vi "RealSense_HelloWorld_On-Chip-Calibration4.vi"() -> ()   [LabVIEW 2017]
doc: "Simple Demo showing how to connect a RealSense Camera to stream COLOR and DEPTH from the stereo camera of a D4xx series camera."
uses:
  healthCheck2.ctl
  libRealSense3.lvlib
panel:
  out "frame time, ms":i64=25
  in  "stop":bool=TRUE
  in  "Use 256x144 for On-Chip Calibration!":u16(ring) items=["256 x 144 @90fps", "424 x 240 @6fps", "424 x 240 @15fps", "424 x 240 @30fps", "424 x 240 @60fps", "424 x 240 @90fps", "480 x 270 @6fps", "480 x 270 @15fps", "480 x 270 @30fps", "480 x 270 @60fps", "480 x 270 @90fps", "640 x 360 @6fps", "640 x 360 @15fps", "640 x 360 @30fps", "640 x 360 @60fps", "640 x 360 @90fps", "640 x 480 @6fps", "640 x 480 @15fps", "640 x 480 @30fps", "640 x 480 @60fps", "640 x 480 @90fps", "848 x 100 @100fps", "848 x 480 @6fps", "848 x 480 @15fps", "848 x 480 @30fps", "848 x 480 @60fps", "848 x 480 @90fps", "1280 x 720 @6fps", "1280 x 720 @15fps", "1280 x 720 @30fps", "1920 x 1080 @15fps", "1920 x 1080 @25fps"]
  in  "Tab Control":T1(tab)
  in  "Depth Presets":T2(ring)=enum."High Accuracy"
  out "Error":bool
  out "Error":bool
  out "AngleX, deg":dbl=-6.76056287473476 format="%.2f"
  out "AngleY, deg":dbl=0.9024890486254136 format="%.2f"
  out "Subpixel, pix":dbl=0.13037986141603491 format="%_3g"
  out "rms error, mm":dbl=1.176758916205707 format="%_3g"
  out "Fill factor (%)":dbl=67.74631076388889 format="%_4g"
  in  "Old / New":bool=TRUE
  in  "SelfCal":bool
  in  "Burn":bool
  out "Healthcheck":T3=0.01235621701925993 scale=0.0..1.8
  in  "laser on/off":bool
  in  "Laser Power,\n mW":sgl=150.0 min=0 max=360
  in  "Gain":sgl=16.0 min=16 max=248
  out "RGB image":picture
  in  "autoexposure":bool
  in  "Exposure,us":sgl=13000.0 min=20 max=1660000
  in  "Tare":bool
  out "Cal Error":string
  in  "Ground Truth, mm":dbl=544.0 format="%.1f"
  out "Measured Z, mm":dbl=543.8435973412348 format="%.1f"
  out "accuracy, %":dbl=-0.02875048874359553 format="%.2f"
  out "Depth map":dbl[][](graph)
  out "OldCalibrationTable":u64=1750951606032
  out "NewCalibrationTable":u64=1750951606320
  in  "Recover Factory Cal.\n(Will stop program)":bool
  in  "Auto Depth Preset\n(5 sec slower)":bool
  in  "A-factor":dbl=0.2
  in  "Calibration Mode":u16(ring) items=["Intrinsic", "Extrinsic"]
  in  "Linux/Windows":u16(ring) items=["Linux+Windows", "Windows Faster"]
  in  "averaging(<30)":u16=10
  in  "Maxstep(5-30)":u16=20
  in  "Accuracy target":u8(ring) items=["Very High (0.025%)", "High (0.05%)", "Medium  (0.1%)", "Low (0.2%)"]
  in  "Self-Calibration Speed":T4(ring)=enum."Fast (Default)"
  out "Camera initialization results":T5={"camera name"="Intel RealSense D435I", "camera S/N"="834412070342", "F/W"="05.12.01.00", "Sensor name"="Stereo Module", "api_version"=23201, "rscontext"=1750951079632, "device_list"=1750948995696, "device count"=1, "Dev out"=1751051540560, "sensor_list"=1750951514688, "sensor count"=3, "Sensor out"=1750945215376}
  out "init error":string="\rNo Error\rNo Error\rNo Error\rNo Error\rNo Error\rNo Error\rNo Error\r\rNo Error\rNo Error"
  out "Config error":string="No Error\rNo Error"
  out "Start Error":string="No Error\rNo Error\rNo Error"
  out "Capture1 Error":string="No Error"
  out "Capture2 error":string="No Error"
  out "Close Error":string="No Error\rNo Error\rNo Error\rNo Error"
  out "release frame error":string="No Error"
  out "Stereo baseline, mm":dbl=49.90683364868164
  out "Intrinsics":T6={"width"=256, "height"=144, "fps"=90, "Profile"=1750952767112, "ppx"=126.45603, "ppy"=71.40294, "fx"=131.32307, "fy"=131.32307, "model"=4}
  # "RealSense Hello World: On-Chip Calibration & Tare"
  # "This demo shows how to connect a RealSense D4xx Stereo Depth Camera, and stream the Monochrome (left) and a DEPTH MAP, and then run on-chip 1. self-calibration to improve depth noise, and 2. Tare to improve accuracy."
  # "MONOCHROME"
  # "ZOOMED (20%) DEPTH MAP"
  # "20-1660000"
  # "Fail-Safe"
  # "16-248"
  # "Point to Flat Wall. Enter the Ground Truth value, and then press Tare. Select \"high accuracy\" Depth Preset before running)"
  # "SELF-CAL \n(DEPTH RMS NOISE)"
  # "Toggle\nCalib."
  # "BURN\n(to ASIC)"
  # "TARE\n(SCALE)"
  # "Point to scene with more than 50% valid depth. Press Self-Cal."
  # "0-360"
  # "Burn after each Tare or Self-Cal."
  # "Common Calibration Settings"
  # "Camera Settings"
  # "For Tare when using \"high accuracy\" depth preset, we recommend using A-factor = 0.2\nFor \"high density\" we recommend A=0.1"
  # "Tare Settings"
  # "Self-Calibration Settings"
  # "The \"speed\" defines the search range. Use \"Fast\" by default, and if you get \"out of range\" error, then try \"slow\""
  # "Use averaging=10, and MaxSteps=20, and Accuracy=Very High for best results. Be sure to use High Accuracy Depth preset or Auto Preset (which will be ~5 seconds slower)"
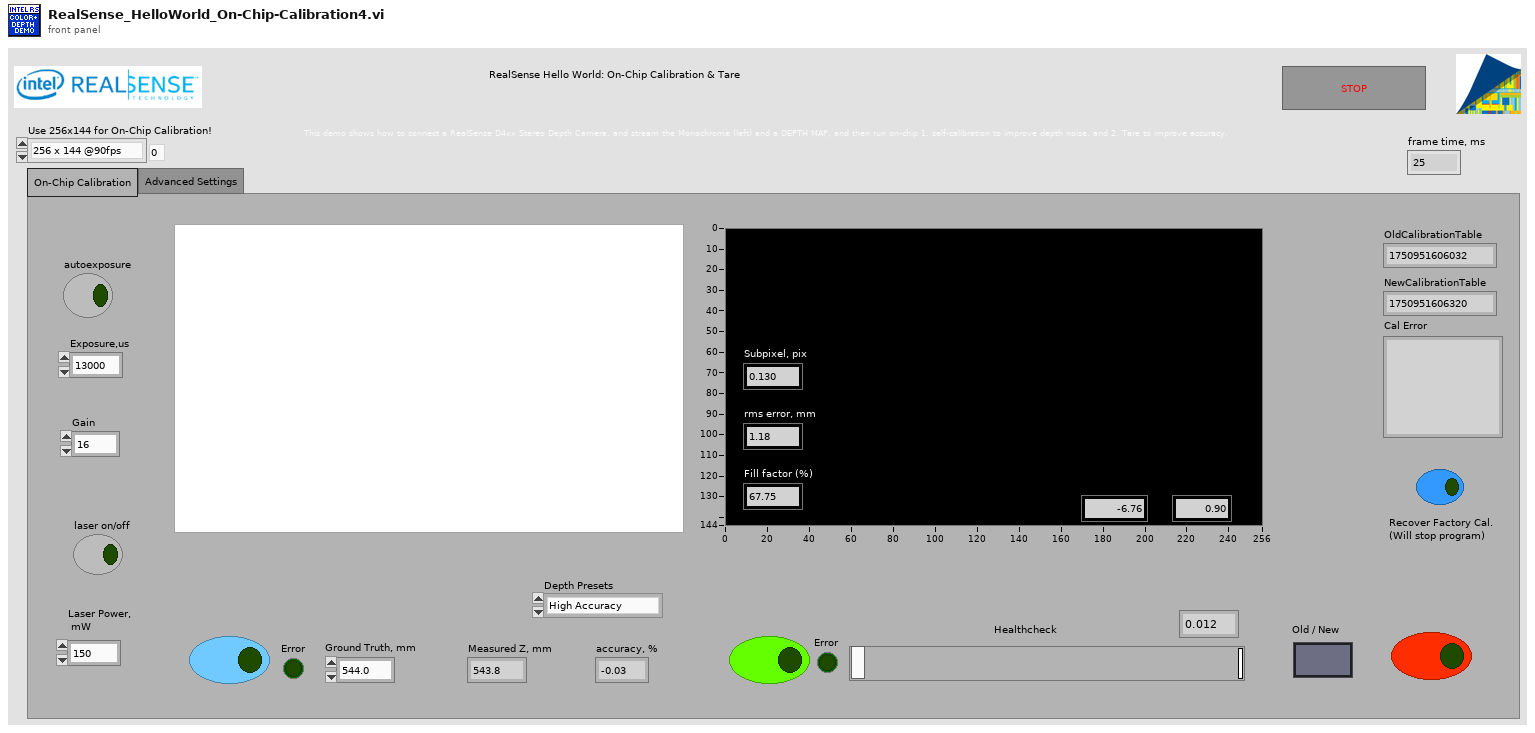
[diagram p1: front panel]
types:
  T1 = enum32{"On-Chip Calibration", "Advanced Settings"}
  T2 = enum16{"Original", "High Density", "Medium Density", "High Accuracy", "Hand", "Short Range", "Flat wall"}
  T3 = typedef "libRealSense3.lvlib/healthCheck2.ctl" = dbl
  T4 = enum16{"Very Fast", "Fast (Default)", "Medium", "Slow", "White Wall"}
  T5 = cluster{"camera name":string, "camera S/N":string, "F/W":string, "Sensor name":string, "api_version":i32, "rscontext":u64, "device_list":u64, "device count":i32, "Dev out":u64, "sensor_list":u64, "sensor count":i32, "Sensor out":u64}
  T6 = cluster{"width":i32, "height":i32, "fps":i32, "Profile":u64, "ppx":sgl, "ppy":sgl, "fx":sgl, "fy":sgl, "model":u32}
  T7 = cluster{"depthUnits":u32, "depthClampMin":u32, "depthClampMax":u32, "disparityMultiplier":u32, "disparityShift":u32}
  T8 = enum16{"Depth", "Color (ext.)", "Color (left) ", "IR Left", "IR Right", "IR Left (Y16)", "IR Right (Y16)"}
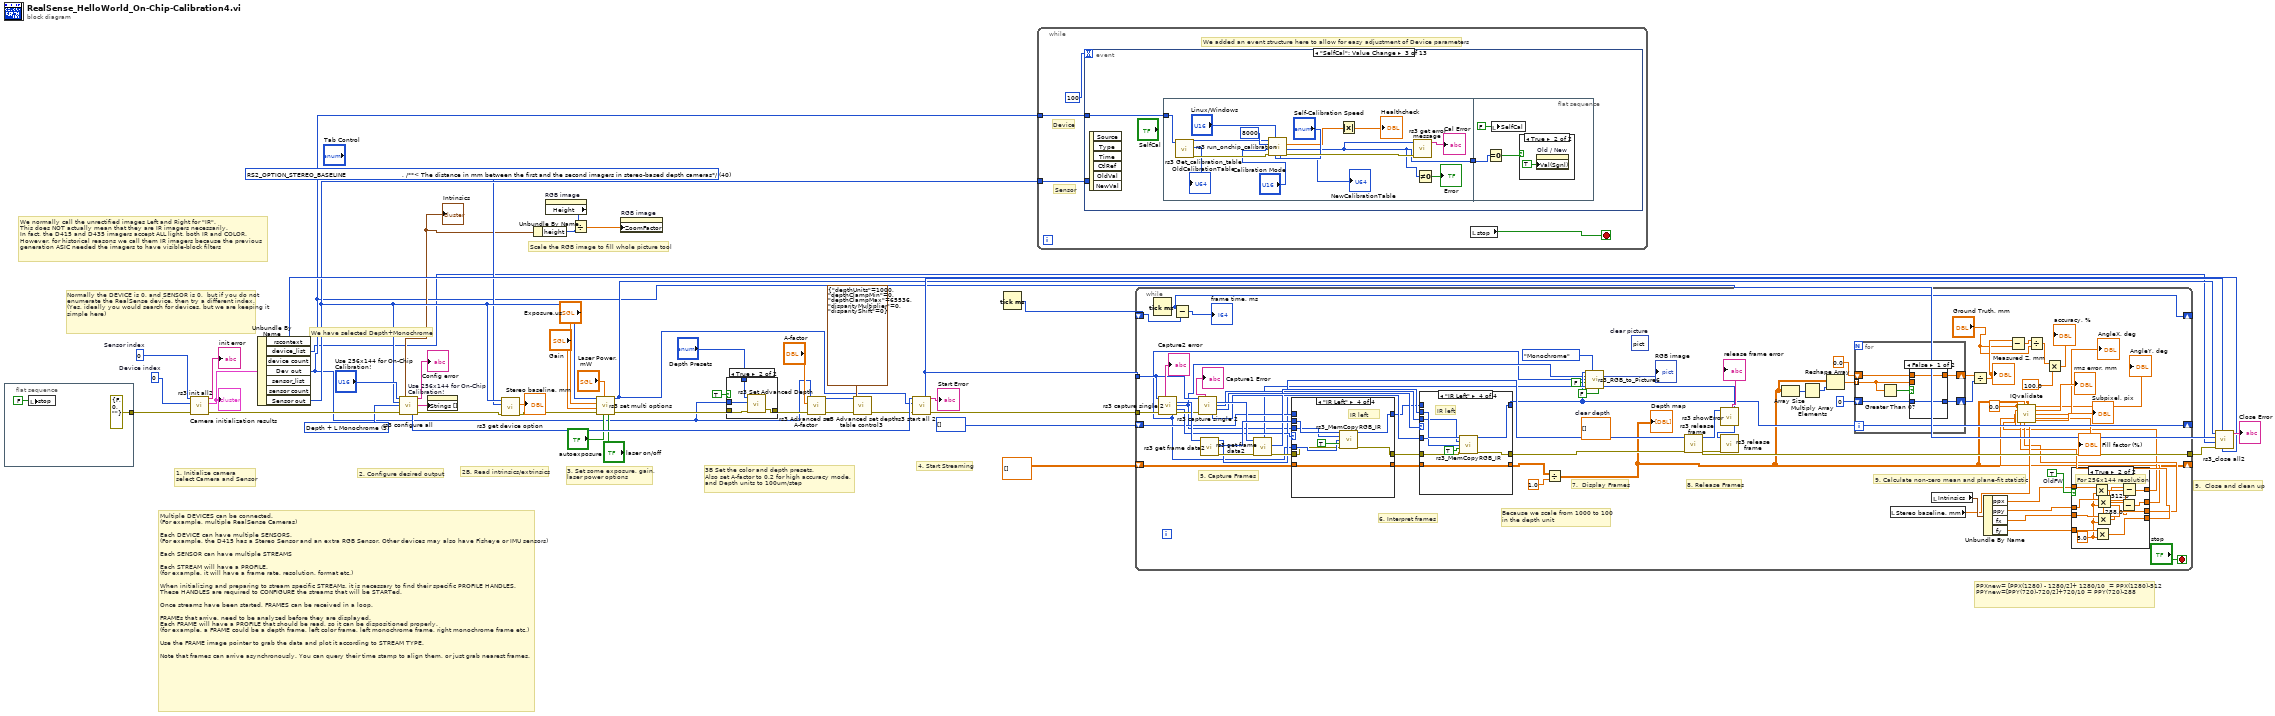
[diagram p0: block diagram]
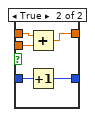
[diagram p4: hidden frame]
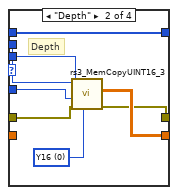
[diagram p6: hidden frame]
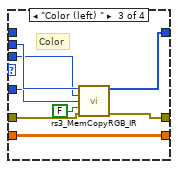
[diagram p7: hidden frame]
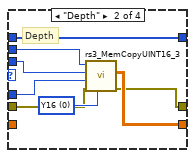
[diagram p9: hidden frame]
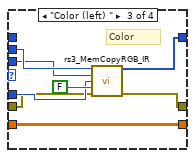
[diagram p10: hidden frame]
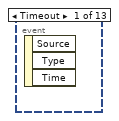
[diagram p11: hidden frame]
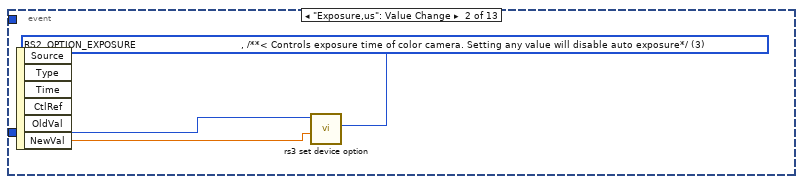
[diagram p12: hidden frame]
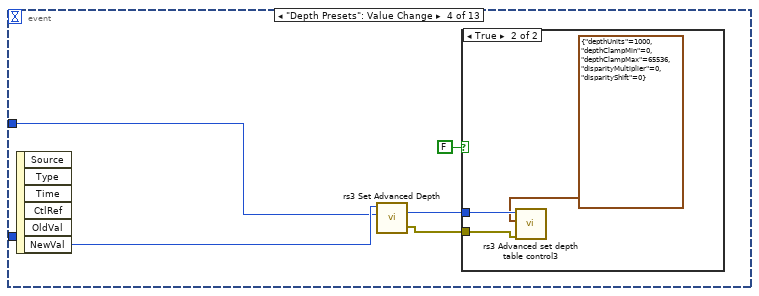
[diagram p14: hidden frame]
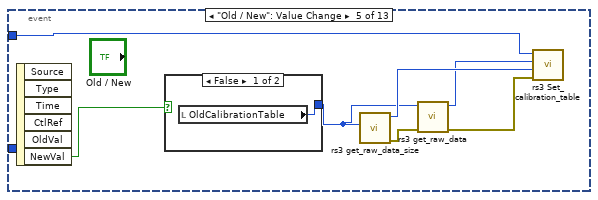
[diagram p16: hidden frame]
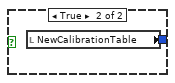
[diagram p17: hidden frame]
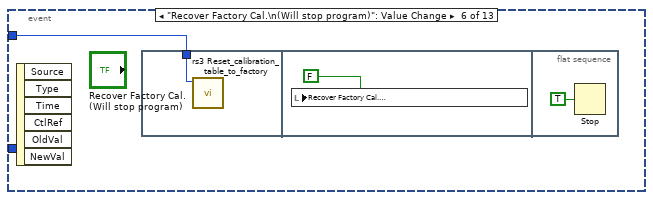
[diagram p18: hidden frame]
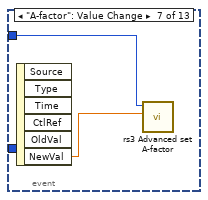
[diagram p19: hidden frame]
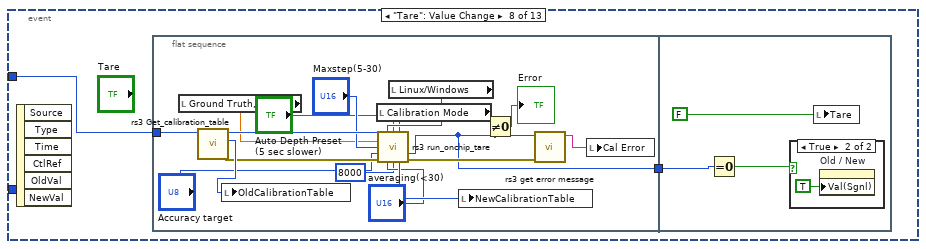
[diagram p20: hidden frame]
diagram:
  w14 = u16 40 items=["    RS2_OPTION_BACKLIGHT_COMPENSATION                     , /**< Enable / disable color backlight compensation*/", "    RS2_OPTION_BRIGHTNESS                                 , /**< Color image brightness*/", "    RS2_OPTION_CONTRAST                                   , /**< Color image contrast*/", "    RS2_OPTION_EXPOSURE                                   , /**< Controls exposure time of color camera. Setting any value will disable auto exposure*/", "    RS2_OPTION_GAIN                                       , /**< Color image gain*/", "    RS2_OPTION_GAMMA                                      , /**< Color image gamma setting*/", "    RS2_OPTION_HUE                                        , /**< Color image hue*/", "    RS2_OPTION_SATURATION                                 , /**< Color image saturation setting*/", "    RS2_OPTION_SHARPNESS                                  , /**< Color image sharpness setting*/", "    RS2_OPTION_WHITE_BALANCE                              , /**< Controls white balance of color image. Setting any value will disable auto white balance*/", "    RS2_OPTION_ENABLE_AUTO_EXPOSURE                       , /**< Enable / disable color image auto-exposure*/", "    RS2_OPTION_ENABLE_AUTO_WHITE_BALANCE                  , /**< Enable / disable color image auto-white-balance*/", "    RS2_OPTION_VISUAL_PRESET                              , /**< Provide access to several recommend sets of option presets for the depth camera */", "    RS2_OPTION_LASER_POWER                                , /**< Power of the F200 / SR300 projector, with 0 meaning projector off*/", "    RS2_OPTION_ACCURACY                                   , /**< Set the number of patterns projected per frame. The higher the accuracy value the more patterns projected. Increasing the number of patterns help to achieve better accuracy. Note that this c", "    RS2_OPTION_MOTION_RANGE                               , /**< Motion vs. Range trade-off, with lower values allowing for better motion sensitivity and higher values allowing for better depth range*/", "    RS2_OPTION_FILTER_OPTION                              , /**< Set the filter to apply to each depth frame. Each one of the filter is optimized per the application requirements*/", "    RS2_OPTION_CONFIDENCE_THRESHOLD                       , /**< The confidence level threshold used by the Depth algorithm pipe to set whether a pixel will get a valid range or will be marked with invalid range*/", "    RS2_OPTION_EMITTER_ENABLED                            , /**< Laser Emitter enabled */", "    RS2_OPTION_FRAMES_QUEUE_SIZE                          , /**< Number of frames the user is allowed to keep per stream. Trying to hold-on to more frames will cause frame-drops.*/", "    RS2_OPTION_TOTAL_FRAME_DROPS                          , /**< Total number of detected frame drops from all streams */", "    RS2_OPTION_AUTO_EXPOSURE_MODE                         , /**< Auto-Exposure modes: Static, Anti-Flicker and Hybrid */", "    RS2_OPTION_POWER_LINE_FREQUENCY                       , /**< Power Line Frequency control for anti-flickering Off/50Hz/60Hz/Auto */", "    RS2_OPTION_ASIC_TEMPERATURE                           , /**< Current Asic Temperature */", "    RS2_OPTION_ERROR_POLLING_ENABLED                      , /**< disable error handling */", "    RS2_OPTION_PROJECTOR_TEMPERATURE                      , /**< Current Projector Temperature */", "    RS2_OPTION_OUTPUT_TRIGGER_ENABLED                     , /**< Enable / disable trigger to be outputed from the camera to any external device on every depth frame */", "    RS2_OPTION_MOTION_MODULE_TEMPERATURE                  , /**< Current Motion-Module Temperature */", "    RS2_OPTION_DEPTH_UNITS                                , /**< Number of meters represented by a single depth unit */", "    RS2_OPTION_ENABLE_MOTION_CORRECTION                   , /**< Enable/Disable automatic correction of the motion data */", "    RS2_OPTION_AUTO_EXPOSURE_PRIORITY                     , /**< Allows sensor to dynamically ajust the frame rate depending on lighting conditions */", "    RS2_OPTION_COLOR_SCHEME                               , /**< Color scheme for data visualization */", "    RS2_OPTION_HISTOGRAM_EQUALIZATION_ENABLED             , /**< Perform histogram equalization post-processing on the depth data */", "    RS2_OPTION_MIN_DISTANCE                               , /**< Minimal distance to the target */", "    RS2_OPTION_MAX_DISTANCE                               , /**< Maximum distance to the target */", "    RS2_OPTION_TEXTURE_SOURCE                             , /**< Texture mapping stream unique ID */", "    RS2_OPTION_FILTER_MAGNITUDE                           , /**< The 2D-filter effect. The specific interpretation is given within the context of the filter */", "    RS2_OPTION_FILTER_SMOOTH_ALPHA                        , /**< 2D-filter parameter controls the weight/radius for smoothing.*/", "    RS2_OPTION_FILTER_SMOOTH_DELTA                        , /**< 2D-filter range/validity threshold*/", "    RS2_OPTION_HOLES_FILL                                 , /**< Enhance depth data post-processing with holes filling where appropriate*/", "    RS2_OPTION_STEREO_BASELINE                            , /**< The distance in mm between the first and the second imagers in stereo-based depth cameras*/", "    RS2_OPTION_AUTO_EXPOSURE_CONVERGE_STEP                , /**< Allows dynamically ajust the converge step value of the target exposure in Auto-Exposure algorithm*/", "    RS2_OPTION_COUNT                                        /**< Number of enumeration values. Not a valid input: intended to be used in for-loops. */"] ("RS Option")
  w20 = u16 5 items=["Depth + Left Color", "Unrectified L + R", "Rectified L + R", "Depth Only", "RGB ext. Only", "Depth + L Monochrome"] ("Stream selection")
  w46 = 0  # Device index
  w45 = 0  # Sensor index
  # "PPXnew= [PPX(1280) - 1280/2]+ 1280/10  = PPX(1280)-512\nPPYnew=[PPY(720)-720/2]+720/10 = PPY(720)-288"
  # "2B. Read intrinsics/extrinsics"
  # "Scale the RGB image to fill whole picture tool"
  # "3B Set the color and depth presets.\nAlso set A-factor to 0.2 for high accuracy mode, \nand Depth units to 100um/step"
  # "We normally call the unrectified images Left and Right for \"IR\". \nThis does NOT actually mean that they are IR imagers necessarily. \nIn fact, the D415 and D435 imagers accept ALL light, both IR and COLOR.\nHowever, for historical reasons we call them IR imagers because the previous generation ASIC needed the imagers to have visible-block filters"
  # "We have selected Depth+Monochrome"
  # "Normally the DEVICE is 0, and SENSOR is 0,  but if you do not enumerate the RealSense device, then try a different index.\n(Yes, ideally you would search for devices, but we are keeping it simple here)"
  # "Multiple DEVICES can be connected. \n(For example, multiple RealSense Cameras)\n\nEach DEVICE can have multiple SENSORS. \n(For example, the D415 has a Stereo Sensor and an extra RGB Sensor. Other devices may also have Fisheye or IMU sensors) \n\nEach SENSOR can have multiple STREAMS\n\nEach STREAM will have a PROFILE. \n(for example, it will have a frame rate, resolution, format etc.)\n\nWhen initializing and preparing to stream specific STREAMs, it is necessary to find their specific PROFILE HANDLES.\nThese HANDLES are required to CONFIGURE the streams that will be STARTed. \n\nOnce streams have been started, FRAMES can be received in a loop. \n \nFRAMEs that arrive, need to be analyzed before they are displayed. \nEach FRAME will have a PROFILE that should be read, so it can be dispositioned properly.\n(for example, a FRAME could be a depth frame, left color frame, left monochrome frame, right monochrome frame etc.)\n\nUse the FRAME image pointer to grab the data and plot it according to STREAM TYPE.\n\nNote that frames can arrive asynchronously. You can query their time stamp to align them, or just grab nearest frames."
  # "9.  Close and clean up"
  # "4. Start Streaming"
  # "3. Set some exposure, gain, \nlaser power options"
  # "2. Configure desired output"
  # "1. Initialize camera\nselect Camera and Sensor"
  n1 = flat-sequence {
    tunnel: [errorcluster {"status"=FALSE, "code"=0, "source"=""} ("error in")] -> w31
    frame #0 {
      n2 = local write "stop"(FALSE ("stop")) -> ()
    }
  }
  n3 = call "rs3 init all2.vi"("error in"=w31, "Select Device"=w46, "Select Sensor"=w45) -> ("error out"=w44:errorcluster, "init results"=w37:T5, "init error"=→"init error":string)  [unwired: 2 in, 4 out]
  "Camera initialization results" <- w37
  n4 = Unbundle By Name(w37) -> ("rscontext"=w36:u64, "device_list"=w1:u64, "Dev out"=w2:u64, "Sensor out"=w15:u64)  [unwired: 3 out]
  n5 = call "rs3 configure all.vi"("Select Resolution"="Use 256x144 for On-Chip Calibration!", "Sensor in"=w15, "Stream selection"=w20, "error in (no error)"=w44) -> ("Output stream L"=w12:T6, "config error"=→"Config error":string, "Output stream"=w32:string[], "Stream Profile Handles"=w43:u64[], "error out"=w17:errorcluster)  [unwired: 2 in, 5 out]
  "Intrinsics" <- w12
  n6 = property on="Use 256x144 for On-Chip Calibration!" class="Ring (strict)"("Strings []"=w32) -> ()  [unwired: 2 in, 2 out]
  n7 = call "rs3 get device option.vi"("error in (no error)"=w17, "RS Option"=w14, "sensor in"=w15) -> ("error out"=w16:errorcluster, "option return"=→"Stereo baseline, mm":dbl)  [unwired: 4 in, 3 out]
  n8 = Unbundle By Name(w12) -> ("height"=w22:i32)
  n9 = property on="RGB image" class="Pict"() -> ("Height"=w21:u32)  [unwired: 2 in, 2 out]
  n10 = Divide(x=w21, y=w22) -> (x/y=w23:dbl)
  n11 = call "rs3 set multi options.vi"("laser on/off"="laser on/off", "autoexposure"="autoexposure", "Laser power, mW (0-360)"="Laser Power,\n mW", "error in (no error)"=w16, "Gain(16-248)"="Gain", "Exposure, us"="Exposure,us", "Sensor in"=w15) -> ("error out"=w19:errorcluster, "Sensor out"=w4:u64)  [unwired: 2 in, 1 out]
  n12 = property on="RGB image" class="Pict"("ZoomFactor"=w23) -> ()  [unwired: 2 in, 2 out]
  n13 = case shown="True" TRUE {
    tunnel: w19 -> [w49 w53]
    tunnel: [w49 w52] -> w11
    tunnel: "Depth Presets" -> [_ w51]
    tunnel: w2 -> [_ w50]
    frame False {
    }
    frame True {
      n14 = call "rs3 Set Advanced Depth.vi"("Depth Presets"=w51, "device in"=w50, "error in (no error)"=w53) -> ("error out"=w52:errorcluster)  [unwired: 1 in, 2 out]
    }
  }
  n15 = call "rs3 Advanced set A-factor.vi"("error in (no error)"=w11, "A-factor (0-0.2)"="A-factor", "device in"=w2) -> ("error out"=w10:errorcluster, "Dev out"=w7:u64)  [unwired: 6 in, 1 out]
  n16 = call "rs3 Advanced set depth table control3.vi"("error in (no error)"=w10, "Depth Table"=T7 {"depthUnits"=1000, "depthClampMin"=0, "depthClampMax"=65536, "disparityMultiplier"=0, "disparityShift"=0}, "device in"=w7) -> ("error out 2"=w9:errorcluster)  [unwired: 6 in, 2 out]
  n17 = call "rs3 start all 2.vi"("error in (no error)"=w9, "Sensor in"=w4, "Stream profile array"=w43) -> ("error out"=w33:errorcluster, "Config Error"=→"Start Error":string, "queue out"=w42:u64)  [unwired: 5 in, 1 out]
  n18 = Tick Count (ms)() -> (millisecond timer value=w6:u32)
  n19 = while {
    tunnel: w2 -> [w56]
    tunnel: w15 -> [w55]
    stop <- w57 stop-if-true
    # "Sensor"
    # "Device"
    # "We added an event structure here to allow for easy adjustment of Device parameters"
    n20 = event shown="[2] \"SelfCal\": Value Change" {
      selector: _ -> [_ _ _ _ _ _ _ _ _ _ _ _ _]
      dyn-events: _ -> [_ _ _ _ _ _ _ _ _ _ _ _ _]
      timeout: 100 -> [_ _ _ _ _ _ _ _ _ _ _ _ _]
      tunnel: w56 -> [_ _ w62 w85 w91 w99 w103 w106 _ _ _ w138 _]
      tunnel: w55 -> [_ w60 _ _ _ _ _ _ w130 w133 w137 _ w154]
      event Timeout {
        n21 = event-data() -> ()  [unwired: 1 in, 3 out]
      }
      event "Exposure,us": Value Change {
        w58 = u16 3 items=["    RS2_OPTION_BACKLIGHT_COMPENSATION                     , /**< Enable / disable color backlight compensation*/", "    RS2_OPTION_BRIGHTNESS                                 , /**< Color image brightness*/", "    RS2_OPTION_CONTRAST                                   , /**< Color image contrast*/", "    RS2_OPTION_EXPOSURE                                   , /**< Controls exposure time of color camera. Setting any value will disable auto exposure*/", "    RS2_OPTION_GAIN                                       , /**< Color image gain*/", "    RS2_OPTION_GAMMA                                      , /**< Color image gamma setting*/", "    RS2_OPTION_HUE                                        , /**< Color image hue*/", "    RS2_OPTION_SATURATION                                 , /**< Color image saturation setting*/", "    RS2_OPTION_SHARPNESS                                  , /**< Color image sharpness setting*/", "    RS2_OPTION_WHITE_BALANCE                              , /**< Controls white balance of color image. Setting any value will disable auto white balance*/", "    RS2_OPTION_ENABLE_AUTO_EXPOSURE                       , /**< Enable / disable color image auto-exposure*/", "    RS2_OPTION_ENABLE_AUTO_WHITE_BALANCE                  , /**< Enable / disable color image auto-white-balance*/", "    RS2_OPTION_VISUAL_PRESET                              , /**< Provide access to several recommend sets of option presets for the depth camera */", "    RS2_OPTION_LASER_POWER                                , /**< Power of the F200 / SR300 projector, with 0 meaning projector off*/", "    RS2_OPTION_ACCURACY                                   , /**< Set the number of patterns projected per frame. The higher the accuracy value the more patterns projected. Increasing the number of patterns help to achieve better accuracy. Note that this c", "    RS2_OPTION_MOTION_RANGE                               , /**< Motion vs. Range trade-off, with lower values allowing for better motion sensitivity and higher values allowing for better depth range*/", "    RS2_OPTION_FILTER_OPTION                              , /**< Set the filter to apply to each depth frame. Each one of the filter is optimized per the application requirements*/", "    RS2_OPTION_CONFIDENCE_THRESHOLD                       , /**< The confidence level threshold used by the Depth algorithm pipe to set whether a pixel will get a valid range or will be marked with invalid range*/", "    RS2_OPTION_EMITTER_ENABLED                            , /**< Laser Emitter enabled */", "    RS2_OPTION_FRAMES_QUEUE_SIZE                          , /**< Number of frames the user is allowed to keep per stream. Trying to hold-on to more frames will cause frame-drops.*/", "    RS2_OPTION_TOTAL_FRAME_DROPS                          , /**< Total number of detected frame drops from all streams */", "    RS2_OPTION_AUTO_EXPOSURE_MODE                         , /**< Auto-Exposure modes: Static, Anti-Flicker and Hybrid */", "    RS2_OPTION_POWER_LINE_FREQUENCY                       , /**< Power Line Frequency control for anti-flickering Off/50Hz/60Hz/Auto */", "    RS2_OPTION_ASIC_TEMPERATURE                           , /**< Current Asic Temperature */", "    RS2_OPTION_ERROR_POLLING_ENABLED                      , /**< disable error handling */", "    RS2_OPTION_PROJECTOR_TEMPERATURE                      , /**< Current Projector Temperature */", "    RS2_OPTION_OUTPUT_TRIGGER_ENABLED                     , /**< Enable / disable trigger to be outputed from the camera to any external device on every depth frame */", "    RS2_OPTION_MOTION_MODULE_TEMPERATURE                  , /**< Current Motion-Module Temperature */", "    RS2_OPTION_DEPTH_UNITS                                , /**< Number of meters represented by a single depth unit */", "    RS2_OPTION_ENABLE_MOTION_CORRECTION                   , /**< Enable/Disable automatic correction of the motion data */", "    RS2_OPTION_AUTO_EXPOSURE_PRIORITY                     , /**< Allows sensor to dynamically ajust the frame rate depending on lighting conditions */", "    RS2_OPTION_COUNT                                      , /**< Number of enumeration values. Not a valid input: intended to be used in for-loops. */"] ("RS Option")
        n22 = event-data() -> ("NewVal"=w59:sgl)  [unwired: 1 in, 5 out]
        n23 = call "rs3 set device option.vi"("value"=w59, "RS Option"=w58, "Sensor in"=w60) -> ()  [unwired: 6 in, 3 out]
      }
      event "SelfCal": Value Change {
        n24 = event-data() -> ()  [unwired: 1 in, 6 out]
        n25 = flat-sequence {
          tunnel: w62 -> [w73]
          tunnel: [w63] -> w61
          tunnel: w61 -> [w79]
          frame #0 {
            n26 = call "rs3 Get_calibration_table.vi"("Device in"=w73) -> ("error out"=w75:errorcluster, "PointerToOldCalibrationTable"=→"OldCalibrationTable":u64, "Device out"=w76:u64)  [unwired: 7 in, 1 out]
            n27 = call "rs3 run_onchip_calibration.vi"("On-Chip Calibration Speed"="Self-Calibration Speed", "Linux/Windows"="Linux/Windows", "error in (no error)"=w75, "On-Chip Calibration Mode"="Calibration Mode", "timeout, ms"=8000, "Device in"=w76) -> ("error out"=w74:errorcluster, "error"=w63:u64, "health-check"=w65:sgl, "PointerToNewCalibrationTable"=→"NewCalibrationTable":u64)  [unwired: 1 in, 1 out]
            n28 = Absolute Value(x=w65) -> (abs(x)=→"Healthcheck":sgl)
            n29 = call "rs3 get error message.vi"("error in (no error)"=w74, "error in"=w63) -> ("error message"=→"Cal Error":string)  [unwired: 7 in, 2 out]
            n30 = Not Equal To 0?(x=w63) -> (x != 0?=→"Error":bool)
          }
          frame #1 {
            n31 = Equal To 0?(x=w79) -> (x = 0?=w78:bool)
            n32 = local write "SelfCal"(FALSE ("SelfCal")) -> ()
            n33 = case shown="True" w78 {
              frame False {
              }
              frame True {
                n34 = property on="Old / New" class="Bool (strict)"("Val(Sgnl)"=TRUE ("Value (Signaling)")) -> ()  [unwired: 2 in, 2 out]
              }
            }
          }
        }
      }
      event "Depth Presets": Value Change {
        n35 = event-data() -> ("NewVal"=w86:T2)  [unwired: 1 in, 5 out]
        n36 = call "rs3 Set Advanced Depth.vi"("Depth Presets"=w86, "device in"=w85) -> ("Dev out"=w84:u64, "error out"=w83:errorcluster)  [unwired: 2 in, 1 out]
        n37 = case shown="True" FALSE {
          tunnel: w84 -> [_ w89]
          tunnel: w83 -> [_ w88]
          frame False {
          }
          frame True {
            n38 = call "rs3 Advanced set depth table control3.vi"("error in (no error)"=w88, "Depth Table"=T7 {"depthUnits"=1000, "depthClampMin"=0, "depthClampMax"=65536, "disparityMultiplier"=0, "disparityShift"=0}, "device in"=w89) -> ()  [unwired: 6 in, 3 out]
          }
        }
      }
      event "Old / New": Value Change {
        n39 = event-data() -> ("NewVal"=w92:bool)  [unwired: 1 in, 5 out]
        n40 = case shown="False" w92 {
          tunnel: [w97 w98] -> w90
          frame False {
            n41 = local read "OldCalibrationTable"() -> (w97:u64)
          }
          frame True {
            n42 = local read "NewCalibrationTable"() -> (w98:u64)
          }
        }
        n43 = call "rs3 get_raw_data_size.vi"("PointToBuffer"=w90) -> ("error out"=w95:errorcluster, "size"=w96:i32)  [unwired: 8 in, 1 out]
        n44 = call "rs3 get_raw_data.vi"("error in (no error)"=w95, "PointerToBuffer"=w90) -> ("error out"=w94:errorcluster, "pointer_to_char_array"=w93:u64)  [unwired: 7 in, 1 out]
        n45 = call "rs3 Set_calibration_table.vi"("error in (no error)"=w94, "calibration_Size"=w96, "PointerToNewCalibrationTable"=w93, "Device in"=w91) -> ()  [unwired: 5 in, 3 out]
      }
      event "Recover Factory Cal.\n(Will stop program)": Value Change {
        n46 = event-data() -> ()  [unwired: 1 in, 6 out]
        n47 = flat-sequence {
          tunnel: w99 -> [w100]
          frame #0 {
            n48 = call "rs3 Reset_calibration_table_to_factory.vi"("Device in"=w100) -> ()  [unwired: 8 in, 3 out]
          }
          frame #1 {
            n49 = local write "Recover Factory Cal.\n(Will stop program)"(FALSE ("Recover Factory Cal.\n(Will stop program)")) -> ()
          }
          frame #2 {
            n50 = Stop(stop? (T)=TRUE) -> ()
          }
        }
      }
      event "A-factor": Value Change {
        n51 = event-data() -> ("NewVal"=w104:dbl)  [unwired: 1 in, 5 out]
        n52 = call "rs3 Advanced set A-factor.vi"("A-factor (0-0.2)"=w104, "device in"=w103) -> ()  [unwired: 7 in, 3 out]
      }
      event "Tare": Value Change {
        n53 = event-data() -> ()  [unwired: 1 in, 6 out]
        n54 = flat-sequence {
          tunnel: w106 -> [w123]
          tunnel: [w108] -> w105
          tunnel: w105 -> [w125]
          frame #0 {
            n55 = local read "Ground Truth, mm"() -> (w110:dbl)
            n56 = call "rs3 Get_calibration_table.vi"("Device in"=w123) -> ("error out"=w118:errorcluster, "PointerToOldCalibrationTable"=w121:u64, "Device out"=w120:u64)  [unwired: 7 in, 1 out]
            n57 = local write "OldCalibrationTable"(w121) -> ()
            n58 = local read "Calibration Mode"() -> (w112:u16)
            n59 = local read "Linux/Windows"() -> (w113:u16)
            n60 = call "rs3 run_onchip_tare.vi"("Device in"=w120, "Linux/Windows"=w113, "Auto Depth Preset\n(5 sec slower)"="Auto Depth Preset\n(5 sec slower)", "On-Chip Calibration Mode"=w112, "ground truth, mm"=w110, "Max step count (5-30)"="Maxstep(5-30)", "accuracy"="Accuracy target", "error in (no error)"=w118, "average step count (1-30)"="averaging(<30)", "timeout ms"=8000) -> ("error"=w108:u64, "PointerToNewCalibrationTable"=w122:u64, "error out"=w119:errorcluster)  [unwired: 2 in, 1 out]
            n61 = local write "NewCalibrationTable"(w122) -> ()
            n62 = Not Equal To 0?(x=w108) -> (x != 0?=→"Error":bool)
            n63 = call "rs3 get error message.vi"("error in (no error)"=w119, "error in"=w108) -> ("error message"=w111:string)  [unwired: 7 in, 2 out]
            n64 = local write "Cal Error"(w111) -> ()
          }
          frame #1 {
            n65 = Equal To 0?(x=w125) -> (x = 0?=w124:bool)
            n66 = case shown="True" w124 {
              frame False {
              }
              frame True {
                n67 = property on="Old / New" class="Bool (strict)"("Val(Sgnl)"=TRUE ("Value (Signaling)")) -> ()  [unwired: 2 in, 2 out]
              }
            }
            n68 = local write "Tare"(FALSE ("Tare")) -> ()
          }
        }
      }
      event "Gain": Value Change {
        w128 = u16 4 items=["    RS2_OPTION_BACKLIGHT_COMPENSATION                     , /**< Enable / disable color backlight compensation*/", "    RS2_OPTION_BRIGHTNESS                                 , /**< Color image brightness*/", "    RS2_OPTION_CONTRAST                                   , /**< Color image contrast*/", "    RS2_OPTION_EXPOSURE                                   , /**< Controls exposure time of color camera. Setting any value will disable auto exposure*/", "    RS2_OPTION_GAIN                                       , /**< Color image gain*/", "    RS2_OPTION_GAMMA                                      , /**< Color image gamma setting*/", "    RS2_OPTION_HUE                                        , /**< Color image hue*/", "    RS2_OPTION_SATURATION                                 , /**< Color image saturation setting*/", "    RS2_OPTION_SHARPNESS                                  , /**< Color image sharpness setting*/", "    RS2_OPTION_WHITE_BALANCE                              , /**< Controls white balance of color image. Setting any value will disable auto white balance*/", "    RS2_OPTION_ENABLE_AUTO_EXPOSURE                       , /**< Enable / disable color image auto-exposure*/", "    RS2_OPTION_ENABLE_AUTO_WHITE_BALANCE                  , /**< Enable / disable color image auto-white-balance*/", "    RS2_OPTION_VISUAL_PRESET                              , /**< Provide access to several recommend sets of option presets for the depth camera */", "    RS2_OPTION_LASER_POWER                                , /**< Power of the F200 / SR300 projector, with 0 meaning projector off*/", "    RS2_OPTION_ACCURACY                                   , /**< Set the number of patterns projected per frame. The higher the accuracy value the more patterns projected. Increasing the number of patterns help to achieve better accuracy. Note that this c", "    RS2_OPTION_MOTION_RANGE                               , /**< Motion vs. Range trade-off, with lower values allowing for better motion sensitivity and higher values allowing for better depth range*/", "    RS2_OPTION_FILTER_OPTION                              , /**< Set the filter to apply to each depth frame. Each one of the filter is optimized per the application requirements*/", "    RS2_OPTION_CONFIDENCE_THRESHOLD                       , /**< The confidence level threshold used by the Depth algorithm pipe to set whether a pixel will get a valid range or will be marked with invalid range*/", "    RS2_OPTION_EMITTER_ENABLED                            , /**< Laser Emitter enabled */", "    RS2_OPTION_FRAMES_QUEUE_SIZE                          , /**< Number of frames the user is allowed to keep per stream. Trying to hold-on to more frames will cause frame-drops.*/", "    RS2_OPTION_TOTAL_FRAME_DROPS                          , /**< Total number of detected frame drops from all streams */", "    RS2_OPTION_AUTO_EXPOSURE_MODE                         , /**< Auto-Exposure modes: Static, Anti-Flicker and Hybrid */", "    RS2_OPTION_POWER_LINE_FREQUENCY                       , /**< Power Line Frequency control for anti-flickering Off/50Hz/60Hz/Auto */", "    RS2_OPTION_ASIC_TEMPERATURE                           , /**< Current Asic Temperature */", "    RS2_OPTION_ERROR_POLLING_ENABLED                      , /**< disable error handling */", "    RS2_OPTION_PROJECTOR_TEMPERATURE                      , /**< Current Projector Temperature */", "    RS2_OPTION_OUTPUT_TRIGGER_ENABLED                     , /**< Enable / disable trigger to be outputed from the camera to any external device on every depth frame */", "    RS2_OPTION_MOTION_MODULE_TEMPERATURE                  , /**< Current Motion-Module Temperature */", "    RS2_OPTION_DEPTH_UNITS                                , /**< Number of meters represented by a single depth unit */", "    RS2_OPTION_ENABLE_MOTION_CORRECTION                   , /**< Enable/Disable automatic correction of the motion data */", "    RS2_OPTION_AUTO_EXPOSURE_PRIORITY                     , /**< Allows sensor to dynamically ajust the frame rate depending on lighting conditions */", "    RS2_OPTION_COUNT                                      , /**< Number of enumeration values. Not a valid input: intended to be used in for-loops. */"] ("RS Option")
        n69 = event-data() -> ("NewVal"=w129:sgl)  [unwired: 1 in, 5 out]
        n70 = call "rs3 set device option.vi"("value"=w129, "RS Option"=w128, "Sensor in"=w130) -> ()  [unwired: 6 in, 3 out]
      }
      event "Laser Power,\n mW": Value Change {
        w131 = u16 13 items=["    RS2_OPTION_BACKLIGHT_COMPENSATION                     , /**< Enable / disable color backlight compensation*/", "    RS2_OPTION_BRIGHTNESS                                 , /**< Color image brightness*/", "    RS2_OPTION_CONTRAST                                   , /**< Color image contrast*/", "    RS2_OPTION_EXPOSURE                                   , /**< Controls exposure time of color camera. Setting any value will disable auto exposure*/", "    RS2_OPTION_GAIN                                       , /**< Color image gain*/", "    RS2_OPTION_GAMMA                                      , /**< Color image gamma setting*/", "    RS2_OPTION_HUE                                        , /**< Color image hue*/", "    RS2_OPTION_SATURATION                                 , /**< Color image saturation setting*/", "    RS2_OPTION_SHARPNESS                                  , /**< Color image sharpness setting*/", "    RS2_OPTION_WHITE_BALANCE                              , /**< Controls white balance of color image. Setting any value will disable auto white balance*/", "    RS2_OPTION_ENABLE_AUTO_EXPOSURE                       , /**< Enable / disable color image auto-exposure*/", "    RS2_OPTION_ENABLE_AUTO_WHITE_BALANCE                  , /**< Enable / disable color image auto-white-balance*/", "    RS2_OPTION_VISUAL_PRESET                              , /**< Provide access to several recommend sets of option presets for the depth camera */", "    RS2_OPTION_LASER_POWER                                , /**< Power of the F200 / SR300 projector, with 0 meaning projector off*/", "    RS2_OPTION_ACCURACY                                   , /**< Set the number of patterns projected per frame. The higher the accuracy value the more patterns projected. Increasing the number of patterns help to achieve better accuracy. Note that this c", "    RS2_OPTION_MOTION_RANGE                               , /**< Motion vs. Range trade-off, with lower values allowing for better motion sensitivity and higher values allowing for better depth range*/", "    RS2_OPTION_FILTER_OPTION                              , /**< Set the filter to apply to each depth frame. Each one of the filter is optimized per the application requirements*/", "    RS2_OPTION_CONFIDENCE_THRESHOLD                       , /**< The confidence level threshold used by the Depth algorithm pipe to set whether a pixel will get a valid range or will be marked with invalid range*/", "    RS2_OPTION_EMITTER_ENABLED                            , /**< Laser Emitter enabled */", "    RS2_OPTION_FRAMES_QUEUE_SIZE                          , /**< Number of frames the user is allowed to keep per stream. Trying to hold-on to more frames will cause frame-drops.*/", "    RS2_OPTION_TOTAL_FRAME_DROPS                          , /**< Total number of detected frame drops from all streams */", "    RS2_OPTION_AUTO_EXPOSURE_MODE                         , /**< Auto-Exposure modes: Static, Anti-Flicker and Hybrid */", "    RS2_OPTION_POWER_LINE_FREQUENCY                       , /**< Power Line Frequency control for anti-flickering Off/50Hz/60Hz/Auto */", "    RS2_OPTION_ASIC_TEMPERATURE                           , /**< Current Asic Temperature */", "    RS2_OPTION_ERROR_POLLING_ENABLED                      , /**< disable error handling */", "    RS2_OPTION_PROJECTOR_TEMPERATURE                      , /**< Current Projector Temperature */", "    RS2_OPTION_OUTPUT_TRIGGER_ENABLED                     , /**< Enable / disable trigger to be outputed from the camera to any external device on every depth frame */", "    RS2_OPTION_MOTION_MODULE_TEMPERATURE                  , /**< Current Motion-Module Temperature */", "    RS2_OPTION_DEPTH_UNITS                                , /**< Number of meters represented by a single depth unit */", "    RS2_OPTION_ENABLE_MOTION_CORRECTION                   , /**< Enable/Disable automatic correction of the motion data */", "    RS2_OPTION_AUTO_EXPOSURE_PRIORITY                     , /**< Allows sensor to dynamically ajust the frame rate depending on lighting conditions */", "    RS2_OPTION_COUNT                                      , /**< Number of enumeration values. Not a valid input: intended to be used in for-loops. */"] ("RS Option")
        n71 = event-data() -> ("NewVal"=w132:sgl)  [unwired: 1 in, 5 out]
        n72 = call "rs3 set device option.vi"("value"=w132, "RS Option"=w131, "Sensor in"=w133) -> ()  [unwired: 6 in, 3 out]
      }
      event "laser on/off": Value Change {
        w136 = u16 18 items=["    RS2_OPTION_BACKLIGHT_COMPENSATION                     , /**< Enable / disable color backlight compensation*/", "    RS2_OPTION_BRIGHTNESS                                 , /**< Color image brightness*/", "    RS2_OPTION_CONTRAST                                   , /**< Color image contrast*/", "    RS2_OPTION_EXPOSURE                                   , /**< Controls exposure time of color camera. Setting any value will disable auto exposure*/", "    RS2_OPTION_GAIN                                       , /**< Color image gain*/", "    RS2_OPTION_GAMMA                                      , /**< Color image gamma setting*/", "    RS2_OPTION_HUE                                        , /**< Color image hue*/", "    RS2_OPTION_SATURATION                                 , /**< Color image saturation setting*/", "    RS2_OPTION_SHARPNESS                                  , /**< Color image sharpness setting*/", "    RS2_OPTION_WHITE_BALANCE                              , /**< Controls white balance of color image. Setting any value will disable auto white balance*/", "    RS2_OPTION_ENABLE_AUTO_EXPOSURE                       , /**< Enable / disable color image auto-exposure*/", "    RS2_OPTION_ENABLE_AUTO_WHITE_BALANCE                  , /**< Enable / disable color image auto-white-balance*/", "    RS2_OPTION_VISUAL_PRESET                              , /**< Provide access to several recommend sets of option presets for the depth camera */", "    RS2_OPTION_LASER_POWER                                , /**< Power of the F200 / SR300 projector, with 0 meaning projector off*/", "    RS2_OPTION_ACCURACY                                   , /**< Set the number of patterns projected per frame. The higher the accuracy value the more patterns projected. Increasing the number of patterns help to achieve better accuracy. Note that this c", "    RS2_OPTION_MOTION_RANGE                               , /**< Motion vs. Range trade-off, with lower values allowing for better motion sensitivity and higher values allowing for better depth range*/", "    RS2_OPTION_FILTER_OPTION                              , /**< Set the filter to apply to each depth frame. Each one of the filter is optimized per the application requirements*/", "    RS2_OPTION_CONFIDENCE_THRESHOLD                       , /**< The confidence level threshold used by the Depth algorithm pipe to set whether a pixel will get a valid range or will be marked with invalid range*/", "    RS2_OPTION_EMITTER_ENABLED                            , /**< Laser Emitter enabled */", "    RS2_OPTION_FRAMES_QUEUE_SIZE                          , /**< Number of frames the user is allowed to keep per stream. Trying to hold-on to more frames will cause frame-drops.*/", "    RS2_OPTION_TOTAL_FRAME_DROPS                          , /**< Total number of detected frame drops from all streams */", "    RS2_OPTION_AUTO_EXPOSURE_MODE                         , /**< Auto-Exposure modes: Static, Anti-Flicker and Hybrid */", "    RS2_OPTION_POWER_LINE_FREQUENCY                       , /**< Power Line Frequency control for anti-flickering Off/50Hz/60Hz/Auto */", "    RS2_OPTION_ASIC_TEMPERATURE                           , /**< Current Asic Temperature */", "    RS2_OPTION_ERROR_POLLING_ENABLED                      , /**< disable error handling */", "    RS2_OPTION_PROJECTOR_TEMPERATURE                      , /**< Current Projector Temperature */", "    RS2_OPTION_OUTPUT_TRIGGER_ENABLED                     , /**< Enable / disable trigger to be outputed from the camera to any external device on every depth frame */", "    RS2_OPTION_MOTION_MODULE_TEMPERATURE                  , /**< Current Motion-Module Temperature */", "    RS2_OPTION_DEPTH_UNITS                                , /**< Number of meters represented by a single depth unit */", "    RS2_OPTION_ENABLE_MOTION_CORRECTION                   , /**< Enable/Disable automatic correction of the motion data */", "    RS2_OPTION_AUTO_EXPOSURE_PRIORITY                     , /**< Allows sensor to dynamically ajust the frame rate depending on lighting conditions */", "    RS2_OPTION_COUNT                                      , /**< Number of enumeration values. Not a valid input: intended to be used in for-loops. */"] ("RS Option")
        n73 = event-data() -> ("NewVal"=w135:bool)  [unwired: 1 in, 5 out]
        n74 = Boolean To (0,1)(Boolean=w135) -> (0, 1=w134:i16)
        n75 = call "rs3 set device option.vi"("value"=w134, "RS Option"=w136, "Sensor in"=w137) -> ()  [unwired: 6 in, 3 out]
      }
      event "Burn": Value Change {
        n76 = event-data() -> ()  [unwired: 1 in, 6 out]
        n77 = flat-sequence {
          tunnel: w138 -> [w143]
          frame #0 {
            w142 = u16 0 items=["Linux (poling)", "Windows (interrupt)"] ("Linux/Windows")
            n78 = call "rs3 Burn_calibration_table.vi"("Device in"=w143) -> ("error out"=w149:errorcluster, "error"=w148:u64)  [unwired: 8 in, 1 out]
            n79 = call "rs3 get error message.vi"("error in (no error)"=w149, "error in"=w148) -> ("error out"=w146:errorcluster, "error message"=w147:string)  [unwired: 7 in, 1 out]
            n80 = local write "Cal Error"(w147) -> ()
            n81 = local read "Calibration Mode"() -> (w140:u16)
            n82 = call "rs3 run_onchip_calibration.vi"("On-Chip Calibration Speed"=T4."Fast (Default)", "Linux/Windows"=w142, "error in (no error)"=w146, "On-Chip Calibration Mode"=w140, "timeout, ms"=4000, "Device in"=w143) -> ("health-check"=w139:sgl, "PointerToNewCalibrationTable"=w145:u64)  [unwired: 1 in, 3 out]
            n83 = local write "NewCalibrationTable"(w145) -> ()
            n84 = local write "Healthcheck"(w139) -> ()
          }
          frame #1 {
            n85 = local write "Burn"(FALSE ("Burn")) -> ()
          }
        }
      }
      event "autoexposure": Value Change {
        w153 = u16 10 items=["    RS2_OPTION_BACKLIGHT_COMPENSATION                     , /**< Enable / disable color backlight compensation*/", "    RS2_OPTION_BRIGHTNESS                                 , /**< Color image brightness*/", "    RS2_OPTION_CONTRAST                                   , /**< Color image contrast*/", "    RS2_OPTION_EXPOSURE                                   , /**< Controls exposure time of color camera. Setting any value will disable auto exposure*/", "    RS2_OPTION_GAIN                                       , /**< Color image gain*/", "    RS2_OPTION_GAMMA                                      , /**< Color image gamma setting*/", "    RS2_OPTION_HUE                                        , /**< Color image hue*/", "    RS2_OPTION_SATURATION                                 , /**< Color image saturation setting*/", "    RS2_OPTION_SHARPNESS                                  , /**< Color image sharpness setting*/", "    RS2_OPTION_WHITE_BALANCE                              , /**< Controls white balance of color image. Setting any value will disable auto white balance*/", "    RS2_OPTION_ENABLE_AUTO_EXPOSURE                       , /**< Enable / disable color image auto-exposure*/", "    RS2_OPTION_ENABLE_AUTO_WHITE_BALANCE                  , /**< Enable / disable color image auto-white-balance*/", "    RS2_OPTION_VISUAL_PRESET                              , /**< Provide access to several recommend sets of option presets for the depth camera */", "    RS2_OPTION_LASER_POWER                                , /**< Power of the F200 / SR300 projector, with 0 meaning projector off*/", "    RS2_OPTION_ACCURACY                                   , /**< Set the number of patterns projected per frame. The higher the accuracy value the more patterns projected. Increasing the number of patterns help to achieve better accuracy. Note that this c", "    RS2_OPTION_MOTION_RANGE                               , /**< Motion vs. Range trade-off, with lower values allowing for better motion sensitivity and higher values allowing for better depth range*/", "    RS2_OPTION_FILTER_OPTION                              , /**< Set the filter to apply to each depth frame. Each one of the filter is optimized per the application requirements*/", "    RS2_OPTION_CONFIDENCE_THRESHOLD                       , /**< The confidence level threshold used by the Depth algorithm pipe to set whether a pixel will get a valid range or will be marked with invalid range*/", "    RS2_OPTION_EMITTER_ENABLED                            , /**< Laser Emitter enabled */", "    RS2_OPTION_FRAMES_QUEUE_SIZE                          , /**< Number of frames the user is allowed to keep per stream. Trying to hold-on to more frames will cause frame-drops.*/", "    RS2_OPTION_TOTAL_FRAME_DROPS                          , /**< Total number of detected frame drops from all streams */", "    RS2_OPTION_AUTO_EXPOSURE_MODE                         , /**< Auto-Exposure modes: Static, Anti-Flicker and Hybrid */", "    RS2_OPTION_POWER_LINE_FREQUENCY                       , /**< Power Line Frequency control for anti-flickering Off/50Hz/60Hz/Auto */", "    RS2_OPTION_ASIC_TEMPERATURE                           , /**< Current Asic Temperature */", "    RS2_OPTION_ERROR_POLLING_ENABLED                      , /**< disable error handling */", "    RS2_OPTION_PROJECTOR_TEMPERATURE                      , /**< Current Projector Temperature */", "    RS2_OPTION_OUTPUT_TRIGGER_ENABLED                     , /**< Enable / disable trigger to be outputed from the camera to any external device on every depth frame */", "    RS2_OPTION_MOTION_MODULE_TEMPERATURE                  , /**< Current Motion-Module Temperature */", "    RS2_OPTION_DEPTH_UNITS                                , /**< Number of meters represented by a single depth unit */", "    RS2_OPTION_ENABLE_MOTION_CORRECTION                   , /**< Enable/Disable automatic correction of the motion data */", "    RS2_OPTION_AUTO_EXPOSURE_PRIORITY                     , /**< Allows sensor to dynamically ajust the frame rate depending on lighting conditions */", "    RS2_OPTION_COUNT                                      , /**< Number of enumeration values. Not a valid input: intended to be used in for-loops. */"] ("RS Option")
        n86 = event-data() -> ("NewVal"=w152:bool)  [unwired: 1 in, 5 out]
        n87 = Boolean To (0,1)(Boolean=w152) -> (0, 1=w151:i16)
        n88 = call "rs3 set device option.vi"("value"=w151, "RS Option"=w153, "Sensor in"=w154) -> ()  [unwired: 6 in, 3 out]
      }
    }
    n89 = local read "stop"() -> (w57:bool)
  }
  n90 = while {
    tunnel: w42 -> [w216]
    tunnel: w33 -> [w225]
    tunnel: [w221] -> w41
    shift-right: [w160] -> _
    shift-left: sgl[][] [] ("2D Array Output") -> [w203]
    shift-right: [w197] -> _
    shift-left: u8[] [] ("Output Array") -> [w201]
    shift-right: [w155] -> _
    shift-left: w6 -> [w157]
    stop <- "stop" stop-if-true
    w171 = TRUE  # OldFW
    w175 = 0.0 ("Ystart")
    (unwired) picture bytes[33]  # clear picture
    (unwired) sgl[][] []  # clear depth
    # "Because we scale from 1000 to 100 \nin the depth unit"
    # "9. Calculate non-zero mean and plane-fit statistic"
    # "8. Release Frames"
    # "7.  Display Frames"
    # "6. Interpret frames"
    # "5. Capture Frames"
    n91 = Tick Count (ms)() -> (millisecond timer value=w155:u32)
    n92 = call "rs3 capture single 2.vi"("queue in"=w216, "error in (no error)"=w225) -> ("Capture Error"=→"Capture2 error":string, "frame out"=w224:u64, "width"=w196:i32, "Stream type"=w204:T8, "height"=w195:i32, "error out"=w217:errorcluster)  [unwired: 2 in, 6 out]
    n93 = Subtract(x=w155, y=w157) -> (x-y=→"frame time, ms":u32)
    n94 = call "rs3 capture single 2.vi"("queue in"=w216, "error in (no error)"=w217) -> ("Capture Error"=→"Capture1 Error":string, "frame out"=w214:u64, "width"=w206:i32, "Stream type"=w208:T8, "height"=w205:i32)  [unwired: 2 in, 7 out]
    n95 = call "rs3 get frame data2.vi"("frame in"=w224) -> ("error out"=w220:errorcluster, "image pointer out"=w223:u64, "Frame out"=w199:u64)  [unwired: 7 in, 1 out]
    n96 = call "rs3 get frame data2.vi"("error in (no error)"=w220, "frame in"=w214) -> ("error out"=w219:errorcluster, "image pointer out"=w207:u64, "Frame out"=w198:u64)  [unwired: 6 in, 1 out]
    n97 = case shown="\"IR Left\"" w204 {
      tunnel: [w285 w290 w297 w305] -> w210
      tunnel: w223 -> [_ w288 w300 w308]
      tunnel: w196 -> [_ w287 w299 w307]
      tunnel: w195 -> [_ w286 w298 w306]
      tunnel: w219 -> [w285 w291 w296 w304]
      tunnel: [w284 w292 w294 w302] -> w202
      tunnel: w203 -> [w284 _ w294 w302]
      tunnel: w201 -> [w283 w289 _ _]
      tunnel: [w283 w289 w295 w303] -> w200
      frame "Color (ext.)", Default {
      }
      frame "Depth" {
        w293 = u16 0 items=["Y16", "Y8"] ("Image format")
        # "Depth"
        n98 = call "rs3_MemCopyUINT16_3.vi"("Image format"=w293, "error in (no error)"=w291, "Depth Y"=w286, "Depth X"=w287, "Zimage pointer"=w288) -> ("error out"=w290:errorcluster, "2D Array Output"=w292:sgl[][])  [unwired: 3 in, 2 out]
      }
      frame "Color (left) " {
        # "Color"
        n99 = call "rs3_MemCopyRGB_IR.vi"("Zimage pointer"=w300, "RGB  X, width"=w299, "RGB Y, height"=w298, "Monochrome(T)/Color(F)"=FALSE ("Grey(T)/Color(F)"), "error in (no error)"=w296) -> ("Output Array"=w295:u8[], "error out"=w297:errorcluster)  [unwired: 8 in, 1 out]
      }
      frame "IR Left" {
        # "IR left"
        n100 = call "rs3_MemCopyRGB_IR.vi"("Zimage pointer"=w308, "RGB  X, width"=w307, "RGB Y, height"=w306, "Monochrome(T)/Color(F)"=TRUE ("Grey(T)/Color(F)"), "error in (no error)"=w304) -> ("Output Array"=w303:u8[], "error out"=w305:errorcluster)  [unwired: 8 in, 1 out]
      }
    }
    n101 = case shown="\"IR Left\"" w208 {
      tunnel: [w258 w263 w272 w280] -> w209
      tunnel: w207 -> [_ w260 w271 w279]
      tunnel: w206 -> [_ w259 w270 w278]
      tunnel: w205 -> [_ w261 w269 w277]
      tunnel: w210 -> [w258 w264 w273 w281]
      tunnel: w202 -> [w257 _ w267 w275]
      tunnel: [w257 w265 w267 w275] -> w162
      tunnel: [w256 w266 w268 w276] -> w197
      tunnel: w200 -> [w256 w266 _ _]
      frame "Color (ext.)", Default {
      }
      frame "Depth" {
        w262 = u16 0 items=["Y16", "Y8"] ("Image format")
        # "Depth"
        n102 = call "rs3_MemCopyUINT16_3.vi"("Image format"=w262, "error in (no error)"=w264, "Depth Y"=w261, "Depth X"=w259, "Zimage pointer"=w260) -> ("error out"=w263:errorcluster, "2D Array Output"=w265:sgl[][])  [unwired: 3 in, 2 out]
      }
      frame "Color (left) " {
        # "Color"
        n103 = call "rs3_MemCopyRGB_IR.vi"("Zimage pointer"=w271, "RGB  X, width"=w270, "RGB Y, height"=w269, "Monochrome(T)/Color(F)"=FALSE ("Grey(T)/Color(F)"), "error in (no error)"=w273) -> ("Output Array"=w268:u8[], "error out"=w272:errorcluster)  [unwired: 8 in, 1 out]
      }
      frame "IR Left" {
        # "IR left"
        n104 = call "rs3_MemCopyRGB_IR.vi"("Zimage pointer"=w279, "RGB  X, width"=w278, "RGB Y, height"=w277, "Monochrome(T)/Color(F)"=TRUE ("Grey(T)/Color(F)"), "error in (no error)"=w281) -> ("Output Array"=w276:u8[], "error out"=w280:errorcluster)  [unwired: 8 in, 1 out]
      }
    }
    n105 = Divide(x=w162, y=1.0) -> (x/y=w160:dbl[][])
    "Depth map" <- w160
    n106 = call "rs3_RGB_to_Picture6.vi"("RGB array"=w197, "Color format"=enum16{"Monochrome", "RGB internal (RGB)"}."Monochrome", "RGB  X, width"=w196, "RGB Y, height"=w195, "AWB"=FALSE, "White Balance"=FALSE) -> ("new picture"=→"RGB image":picture)  [unwired: 8 in, 1 out]
    n107 = call "rs3 release frame.vi"("error in (no error)"=w209, "Frame"=w199) -> ("error out"=w222:errorcluster, "error"=w213:u64)  [unwired: 8 in]
    n108 = call "rs3 showError.vi"("error"=w213) -> ("Error summary"=→"release frame error":string)  [unwired: 6 in, 4 out]
    n109 = call "rs3 release frame.vi"("error in (no error)"=w222, "Frame"=w198) -> ("error out"=w221:errorcluster)  [unwired: 8 in, 1 out]
    n110 = Array Size(array=w160) -> (size(s)=w190:i32[])
    n111 = Multiply Array Elements(1:w190) -> (0:w189:i32)
    n112 = Reshape Array(w160, w189) -> (w188:dbl[])
    n113 = for {
      tunnel: w188 -> [w246] mode=indexing
      shift-right: [w245] -> w185
      shift-left: 0.0 -> [w247]
      shift-right: [w243] -> w184
      shift-left: u64 0 -> [w244]
      n114 = Greater Than 0?(x=w246) -> (x > 0?=w248:bool)
      n115 = case shown="False" w248 {
        tunnel: w247 -> [w250 w255]
        tunnel: w246 -> [_ w254]
        tunnel: [w250 w253] -> w245
        tunnel: w244 -> [w249 w252]
        tunnel: [w249 w251] -> w243
        frame False {
        }
        frame True {
          n116 = Add(x=w255, y=w254) -> (x+y=w253:dbl)
          n117 = Increment(x=w252) -> (x+1=w251:u64)
        }
      }
    }
    n118 = local read "Stereo baseline, mm"() -> (w176:dbl)
    n119 = local read "Intrinsics"() -> (w177:T6)
    n120 = Divide(x=w185, y=w184) -> (x/y=w183:dbl)
    "Measured Z, mm" <- w183
    n121 = Unbundle By Name(w177) -> ("ppx"=w167:sgl, "ppy"=w168:sgl, "fx"=w170:sgl, "fy"=w169:sgl)
    n122 = Subtract(x=w183, y="Ground Truth, mm") -> (x-y=w182:dbl)
    n123 = Divide(x=w182, y="Ground Truth, mm") -> (x/y=w180:dbl)
    n124 = Multiply(x=w180, y=100.0) -> (x*y=→"accuracy, %":dbl)
    n125 = case shown="True" w171 {
      tunnel: w170 -> [w229 w241]
      tunnel: w169 -> [w228 w242]
      tunnel: w168 -> [w226 w240]
      tunnel: w167 -> [w227 w239]
      tunnel: [w228 w237] -> w166
      tunnel: [w229 w236] -> w165
      tunnel: [w227 w233] -> w164
      tunnel: [w226 w230] -> w163
      frame False {
      }
      frame True {
        w238 = sgl 5.0 ("y")
        # "For 256x144 resolution"
        n126 = Multiply(x=w239, y=w238) -> (x*y=w235:sgl)
        n127 = Multiply(x=w242, y=w238) -> (x*y=w237:sgl)
        n128 = Multiply(x=w240, y=w238) -> (x*y=w231:sgl)
        n129 = Multiply(x=w241, y=w238) -> (x*y=w236:sgl)
        n130 = Subtract(x=w231, y=sgl 288.0) -> (x-y=w230:sgl)
        n131 = Subtract(x=w235, y=sgl 512.0) -> (x-y=w233:sgl)
      }
    }
    n132 = call "IQvalidate.vi"("Ystart"=w175, "Xstart"=w175, "Depth Map"=w160, "baseline, mm"=w176, "ppx"=w164, "ppy"=w163, "fy"=w166, "fx"=w165) -> ("AngleY"=→"AngleY, deg":dbl, "rms error value, mm"=→"rms error, mm":dbl, "AngleX"=→"AngleX, deg":dbl, "Fill factor (%) \n(new)"=→"Fill factor (%)":dbl, "Subpixel, pix"=→"Subpixel, pix":dbl)  [unwired: 3 out]
  }
  n133 = call "rs3_close all2.vi"("rscontext"=w36, "queue in"=w42, "error in (no error)"=w41, "device_list"=w1, "Dev in"=w2, "Sensor in"=w4) -> ("Close Error"=→"Close Error":string)  [unwired: 4 in, 1 out]
